vi "Ec.vi"(1 "Test Section Length (Lts)":dbl, 2 "Equivalent Collector Radius (Rc)":dbl, 3 "Turn-table Centre (Xm)":dbl, 4 "Wake Blockage Factor (Ew)":dbl) -> (0 "Collector Blockage Correction (Ec)":dbl)   [LabVIEW 2017]
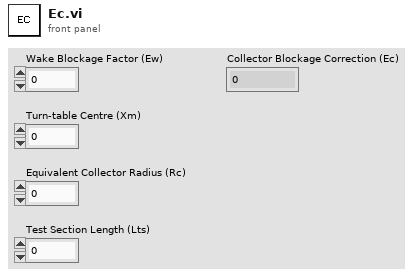
[diagram p1: front panel]
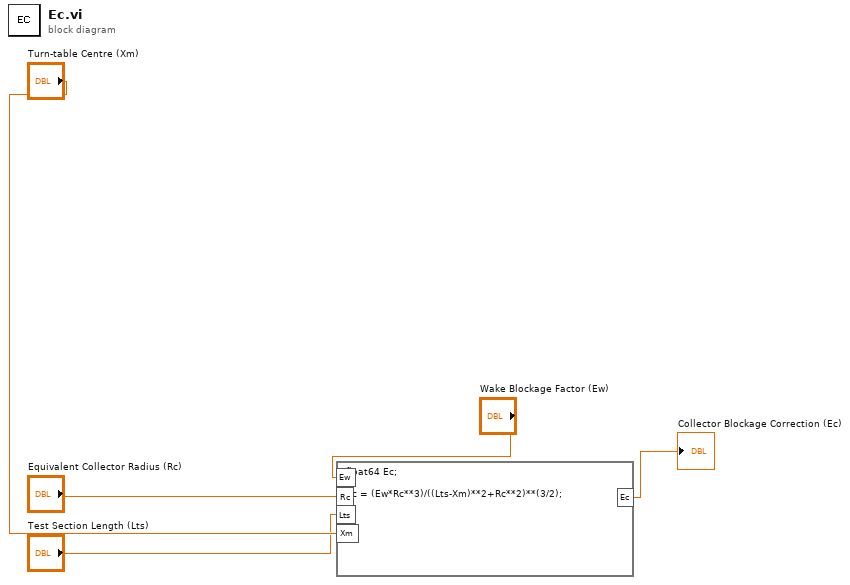
[diagram p0: block diagram]
diagram:
  n1 = formula code="float64 Ec;\n\nEc = (Ew*Rc**3)/((Lts-Xm)**2+Rc**2)**(3/2);"("Ew"="Wake Blockage Factor (Ew)", "Rc"="Equivalent Collector Radius (Rc)", "Lts"="Test Section Length (Lts)", "Xm"="Turn-table Centre (Xm)") -> ("Ec"=→"Collector Blockage Correction (Ec)":dbl)
